vi "Example.vi"() -> ()   [LabVIEW 2013]
uses:
  Client/Client.lvclass/Client.ctl
  Client/Client.lvclass
  Control Packets/PUBLISH/PUBLISH.lvclass
  MQTT_Base/MQTT_Base.lvclass
panel:
  out "value":i32
  out "Subscription Event":variant
  out "Topic":string
  in  "stop":bool
  out "Published":bool
  in  "error in (no error)":errorcluster
  out "error out":errorcluster
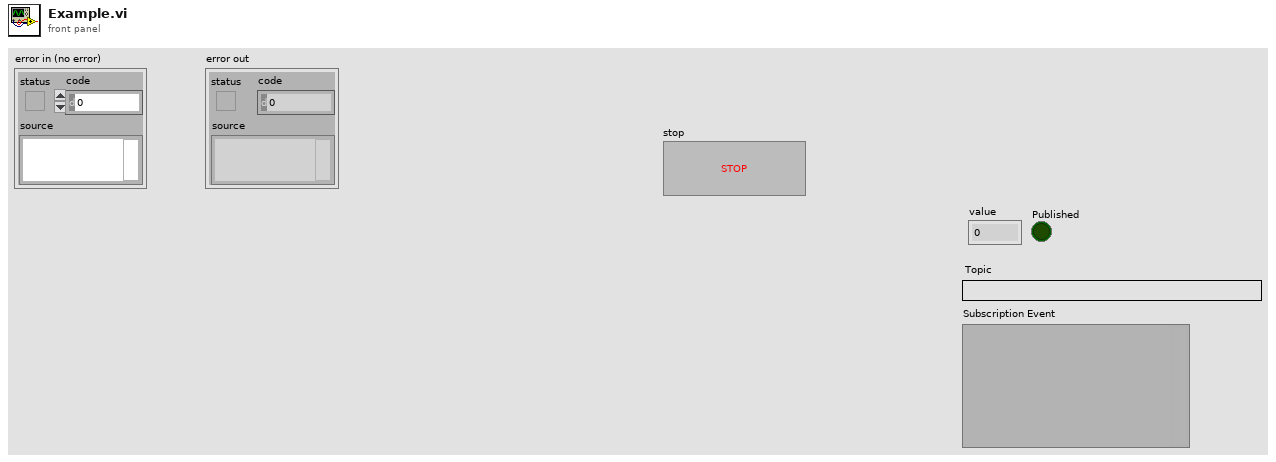
[diagram p1: front panel]
types:
  T1 = typedef "MQTT Server.lvlib/Client.lvclass/Public Events -- cluster.ctl" = cluster{"Connection Status":refnum<user-event>, "Connected":refnum<user-event>, "Application Message":refnum<user-event>}
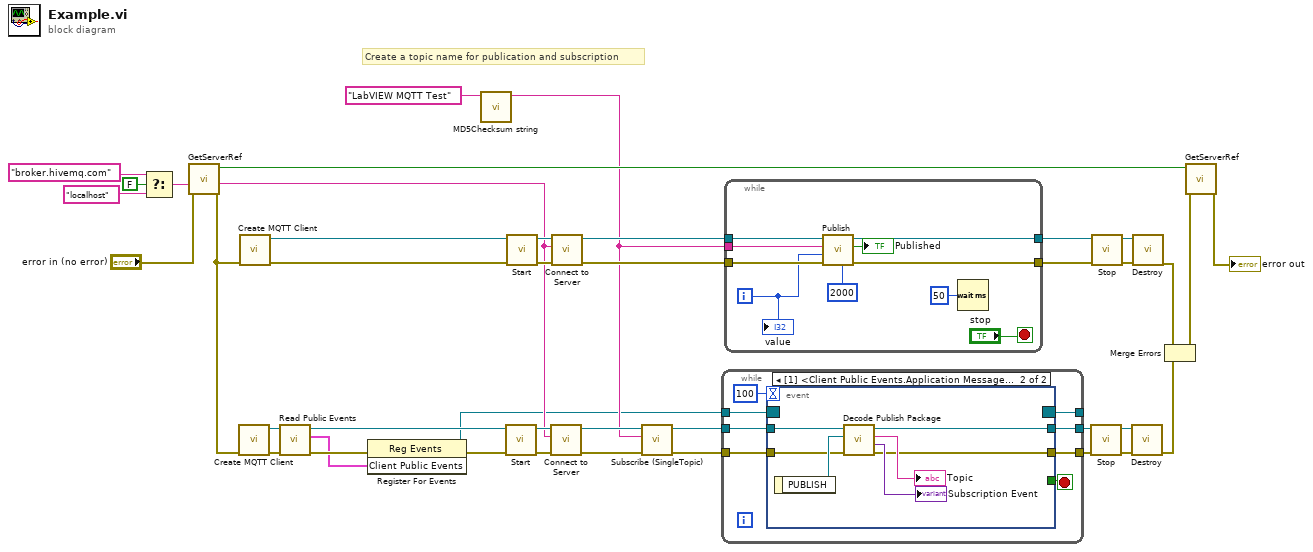
[diagram p0: block diagram]
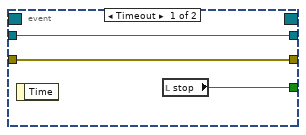
[diagram p2: hidden frame]
diagram:
  # "Create a topic name for publication and subscription"
  n1 = Select(t="broker.hivemq.com" ("address (localhost)"), s=FALSE, f="localhost" ("address (localhost)")) -> (s? t:f=w28:string)
  n2 = call "GetServerRef.vi"("error in"="error in (no error)", "address (localhost)"=w28) -> ("error out"=w16:errorcluster, "Server address"=w17:string, "Created"=w41:bool)  [unwired: 6 in, 1 out]
  n3 = call "Create MQTT Client.vi"("error in (no error)"=w16) -> ("error out"=w5:errorcluster, "Client out"=w7:refnum<class "Client.lvclass">)  [unwired: 9 in]
  n4 = call "Create MQTT Client.vi"("error in (no error)"=w16) -> ("error out"=w35:errorcluster, "Client out"=w36:refnum<class "Client.lvclass">)  [unwired: 9 in]
  n5 = call "Read Public Events.vi"("error in (no error)"=w5, "Client in"=w7) -> ("error out"=w4:errorcluster, "Client Public Events"=w2:T1, "Client out"=w6:refnum<class "Client.lvclass">)  [unwired: 7 in]
  n6 = register-events(error in=w4, w2) -> (reference out=w1:refnum<event-registration>, error out=w3:errorcluster)  [unwired: 1 in]
  n7 = call <vilib>:"MD5Checksum string.vi"("Message String"="LabVIEW MQTT Test" ("Topic Name (empty: Payload name)")) -> ("MD5 message-digest"=w11:string)  [unwired: 10 in]
  n8 = call "Start.vi"("error in (no error)"=w3, "MQTT_Base in"=w6) -> ("error out"=w19:errorcluster, "MQTT_Base out"=w18:refnum<class "Client.lvclass">)  [unwired: 7 in, 1 out]
  n9 = call "Start.vi"("error in (no error)"=w35, "MQTT_Base in"=w36) -> ("error out"=w38:errorcluster, "MQTT_Base out"=w39:refnum<class "Client.lvclass">)  [unwired: 7 in, 1 out]
  n10 = call "Connect to Server.vi"("error in (no error)"=w19, "address (localhost)"=w17, "Client in"=w18) -> ("error out"=w13:errorcluster, "Client out"=w15:refnum<class "Client.lvclass">)  [unwired: 5 in, 2 out]
  n11 = call "Connect to Server.vi"("error in (no error)"=w38, "address (localhost)"=w17, "Client in"=w39) -> ("error out"=w32:errorcluster, "Client out"=w33:refnum<class "Client.lvclass">)  [unwired: 5 in, 2 out]
  n12 = call "Subscribe (SingleTopic).vi"("error in (no error)"=w13, "Topic Filter"=w11, "MQTT_Base in"=w15) -> ("error out"=w12:errorcluster, "MQTT_Base out"=w14:refnum<class "Client.lvclass">)  [unwired: 7 in]
  n13 = while {
    tunnel: w14 -> [w44]
    tunnel: w12 -> [w42]
    tunnel: [w45] -> w22
    tunnel: [w43] -> w23
    tunnel: w1 -> [w47]
    tunnel: [w46] -> _
    stop <- w48 stop-if-true
    n14 = event shown="[1] <Client Public Events.Application Message>: User Event" {
      selector: w47 -> [_ _]
      dyn-events: [_ _] -> w46
      timeout: 100 -> [_ _]
      tunnel: [w52 _] -> w48
      tunnel: w44 -> [w51 w58]
      tunnel: [w51 w55] -> w45
      tunnel: [w50 w53] -> w43
      tunnel: w42 -> [w50 w54]
      event Timeout {
        n15 = event-data() -> ()  [unwired: 1 in, 1 out]
        n16 = local read "stop"() -> (w52:bool)
      }
      event User Event {
        n17 = event-data() -> ("PUBLISH"=w59:refnum<class "PUBLISH.lvclass">)  [unwired: 1 in]
        n18 = call "Decode Publish Package.vi"("error in (no error)"=w54, "PUBLISH in"=w59, "MQTT_Base in"=w58) -> ("error out"=w53:errorcluster, "Payload"=→"Subscription Event":variant, "Topic"=→"Topic":string, "MQTT_Base out"=w55:refnum<class "Client.lvclass">)  [unwired: 5 in]
      }
    }
  }
  n19 = while {
    tunnel: w33 -> [w69]
    tunnel: w32 -> [w68]
    tunnel: [w66] -> w27
    tunnel: [w65] -> w26
    tunnel: w11 -> [w63]
    i -> [w60]
    stop <- "stop" stop-if-true
    n20 = call "Publish.vi"("timeout (1000ms)"=2000, "error in (no error)"=w68, "Payload"=w60, "Topic Name (empty: Payload name)"=w63, "Client in"=w69) -> ("error out"=w65:errorcluster, "Published"=→"Published":bool, "Client out"=w66:refnum<class "Client.lvclass">)  [unwired: 4 in]
    n21 = Wait (ms)(milliseconds to wait=u32 50) -> ()  [unwired: 1 out]
    "value" <- w60
  }
  n22 = call "Stop.vi"("error in (no error)"=w23, "MQTT_Base in"=w22) -> ("error out"=w21:errorcluster, "MQTT_Base out"=w20:refnum<class "Client.lvclass">)  [unwired: 7 in, 1 out]
  n23 = call "Stop.vi"("error in (no error)"=w26, "MQTT_Base in"=w27) -> ("error out"=w34:errorcluster, "MQTT_Base out"=w37:refnum<class "Client.lvclass">)  [unwired: 7 in, 1 out]
  n24 = call-dynamic "Destroy.vi"("error in (no error)"=w21, "Client in"=w20) -> ("error out"=w10:errorcluster)  [unwired: 8 in, 1 out]
  n25 = call-dynamic "Destroy.vi"("error in (no error)"=w34, "Client in"=w37) -> ("error out"=w9:errorcluster)  [unwired: 8 in, 1 out]
  n26 = Merge Errors(w9, w10) -> (w8:errorcluster)
  n27 = call "GetServerRef.vi"("error in"=w8, "Destroy (F)"=w41) -> ("error out"=→"error out":errorcluster)  [unwired: 6 in, 3 out]
